vi "ReadTemp2.vi"(0 "VISA Refnum in":refnum<visa-resource-name>, 2 "Address":u8, 3 "error in (no error)":errorcluster) -> (1 "Temp":i16, 6 "VISA Refnum out":refnum<visa-resource-name>, 7 "Valid":bool, 10 "error out":errorcluster)   [LabVIEW 2015, in "Ion Motion Roboclaw.lvlib"]
uses:
  <instrlib>/Ion Motion Roboclaw/Ion Motion Roboclaw.lvlib
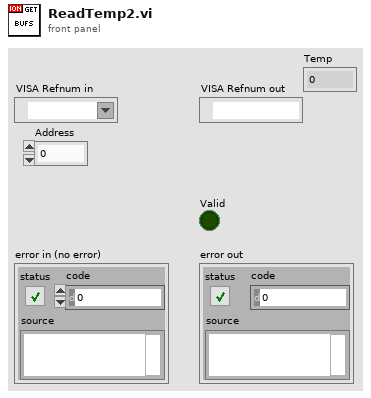
[diagram p1: front panel]
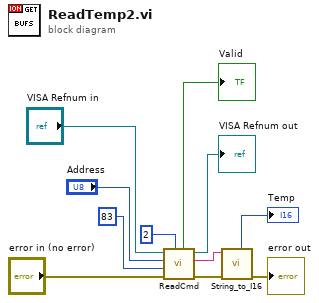
[diagram p0: block diagram]
diagram:
  n1 = call <instrlib>:"ReadCmd.vi"("Read Count"=u32 2, "error in (no error)"="error in (no error)", "Cmd"=u8 83, "Address"="Address", "VISA Refnum in"="VISA Refnum in") -> ("error out"=w3:errorcluster, "Output"=w2:string, "VISA Refnum out"=→"VISA Refnum out":refnum<visa-resource-name>, "Valid"=→"Valid":bool)  [unwired: 3 in]
  n2 = call <instrlib>:"String_to_I16.vi"("error in (no error)"=w3, "String"=w2) -> ("error out"=→"error out":errorcluster, "number"=→"Temp":i16)  [unwired: 5 in, 1 out]
